vi "CronState.vi"(10 "new value":bool, 11 "cron id":string) -> (3 "previous":bool)   [LabVIEW 2017, in "CronScheduler.lvlib"]
uses:
  <vilib>/addons/InsightCM/Utilities/CronScheduler/CronScheduler.lvlib
  <vilib>/addons/InsightCM/Utilities/PropertyHelpers/PropertyHelpers.lvlib
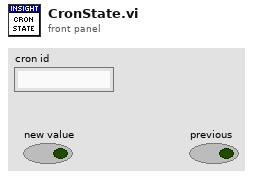
[diagram p1: front panel]
types:
  T1 = typedef "KeyValuePair.ctl" = cluster{"Key":string, "Value":string}
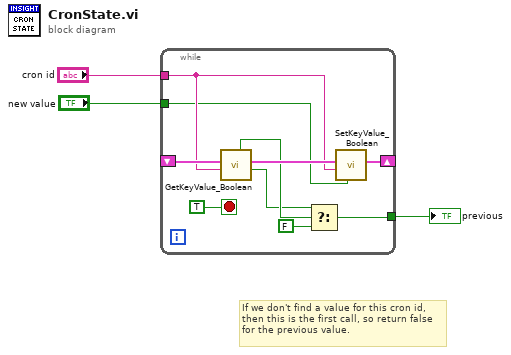
[diagram p0: block diagram]
diagram:
  # "If we don't find a value for this cron id,\nthen this is the first call, so return false\nfor the previous value."
  n1 = while {
    tunnel: "cron id" -> [w10]
    shift-right: [w9] -> _
    shift-left: _ -> [w12]
    tunnel: "new value" -> [w8]
    tunnel: [w5] -> w1
    stop <- TRUE stop-if-true
    n2 = call <vilib>:"GetKeyValue_Boolean.vi"("key"=w10, "key value pairs"=w12) -> ("value"=w6:bool, "key value pairs out"=w11:T1[], "found"=w7:bool)  [unwired: 7 in]
    n3 = Select(t=w6, s=w7, f=FALSE) -> (s? t:f=w5:bool)
    n4 = call <vilib>:"SetKeyValue_Boolean.vi"("value"=w8, "key"=w10, "key value pairs"=w11) -> ("key value pairs out"=w9:T1[])  [unwired: 8 in]
  }
  "previous" <- w1
